vi "Conditional_Timer.vi"(1 "Suppress?":bool=TRUE, 2 "milliseconds to wait":u32=500) -> ()   [LabVIEW 2016]
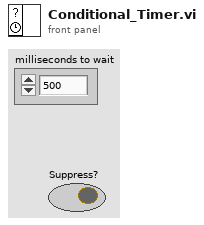
[diagram p1: front panel]
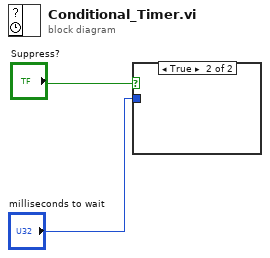
[diagram p0: block diagram]
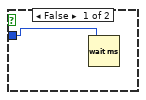
[diagram p2: hidden frame]
diagram:
  n1 = case shown="True" "Suppress?" {
    tunnel: "milliseconds to wait" -> [w3 _]
    frame False {
      n2 = Wait (ms)(milliseconds to wait=w3) -> ()  [unwired: 1 out]
    }
    frame True {
    }
  }
